vi "Trigger Instrument View.vi"(8 "error in (no error)":errorcluster, 9 "New Value":u16, 10 "Old Value":u16, 11 "Instruments in":refnum<class "Instruments.lvclass">) -> (0 "error out":errorcluster, 3 "Instruments out":refnum<class "Instruments.lvclass">)   [LabVIEW 2023, in "Instruments.lvlib" / "Instruments.lvclass"]
doc: "<b>Trigger Instrument View</b>\nThis generates a change instrument event, changing what instrument is displayed in the panel, allowing a station to support many instruments with few display panes."
uses:
  Library/Instruments.lvclass
  Library/Instruments.lvclass/Instruments.ctl
  builds/Framework/Engine.lvlibp/Engine/Library/Engine.lvclass
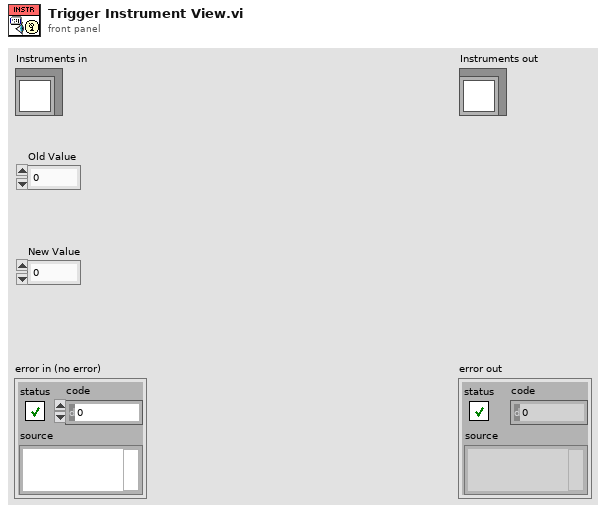
[diagram p1: front panel]
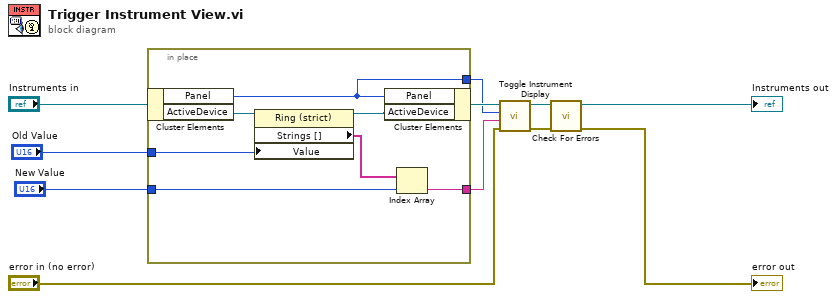
[diagram p0: block diagram]
diagram:
  n1 = in-place {
    in-place-border: "Old Value" -> [w15]
    in-place-border: "New Value" -> [w14]
    in-place-border: [w13] -> w2
    in-place-border: [w12] -> w1
    n2 = in-place-cluster #1("Instruments in") -> ("Panel"=w13:i32, "ActiveDevice"=w18:refnum<vi>)
    n3 = property class="Ring (strict)"(reference=w18, "Value"=w15) -> (reference out=w17:refnum<vi>, "Strings []"=w16:string[])  [unwired: 1 in, 1 out]
    n4 = in-place-cluster #1("Panel"=w13, "ActiveDevice"=w17) -> (w7:refnum<class "Instruments.lvclass">)
    n5 = Index Array(array=w16, index=w14) -> (element=w12:string)
  }
  n6 = call "Toggle Instrument Display.vi"("error in (no error)"="error in (no error)", "Instrument"=w1, "Panel"=w2, "Engine in"=w7) -> ("error out"=w11:errorcluster, "Engine out"=w10:refnum<class "Instruments.lvclass">)  [unwired: 6 in]
  n7 = call "Check For Errors.vi"("error in"=w11, "Engine in"=w10) -> ("error out"=→"error out":errorcluster, "Engine out"=→"Instruments out":refnum<class "Instruments.lvclass">)  [unwired: 8 in]
